vi "game.vi"() -> ()   [LabVIEW 2016]
panel:
  in  "ModeIsSetting":bool=TRUE
  in  "Tab Control":enum32{"Game", "Settings", "How to Play"}(tab)
  out "Target LED Ready":bool
  out "Current Player":string
  out "?":bool[](array[boolean])
  out "?":bool[](array[boolean])
  out "Players":string[](array[string])
  out "Scores":i32[](array[numeric])
  out "Current Player":i32
  out "Current LED":i32
  out "LED Ready":bool
  out "Target LED":i32
  out "player ready":bool=TRUE
  in  "stop":bool
  in  "RESET":bool
  out "Score":string
  in  "current duration":u32
  in  "Start The Game":bool
  in  "Game Mode":enum16{"Easy", "Hard", "Very Hard"}(ring)
  in  "LED count":i32=10
  in  "starting LED\nduration":u32=100
  in  "Player count":i32=2
  in  "Player prefix":string="Player"
  in  "duration decrease":u32=20
  in  "min duration":u32=60
  in  "Target Led duration":i32=1000
  out "Blank LEDs":bool[](array[boolean])
  # "L  E  D     G  A  M  E  !"
  # "Game Settings"
  # "H o w    t o    P l a y    ?"
  # "1 - Set the parameters in the settings tab as you wish\n\n2 - By clicking on the stop button you can stop the circle LED in the red state. The rectangle red LED shows on which led you should click on the stop button.\n\n3 - The more closer you stop the red circle LED to red rectangle LED, the more points you achieve to gain.\n\n4 - Be carefull, as the game moves on, the the LEDs will start to turn on and off more quickly according to the settings you choose.\n\n5 - Modes\nEasy: The target LED does not move.\nHard: The target LED also moves with the duration you set in the settings tab.\nVery Hard: The target LED moves randomly, being talented is not enough you should also be lucky ! \n\n\n                                                           Have Fun !"
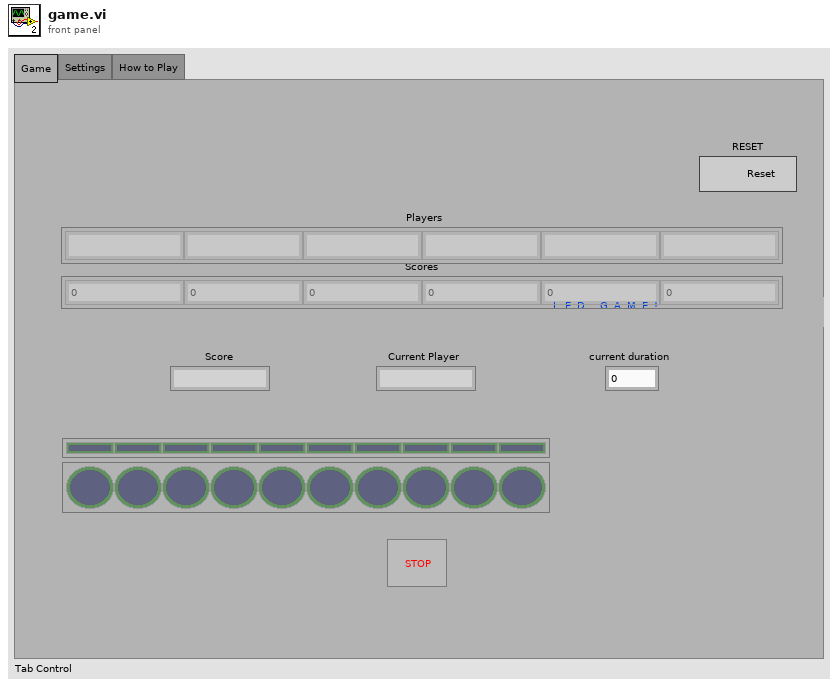
[diagram p1: front panel]
types:
  T1 = enum8{"Enabled", "Disabled", "Disabled and Grayed Out"}
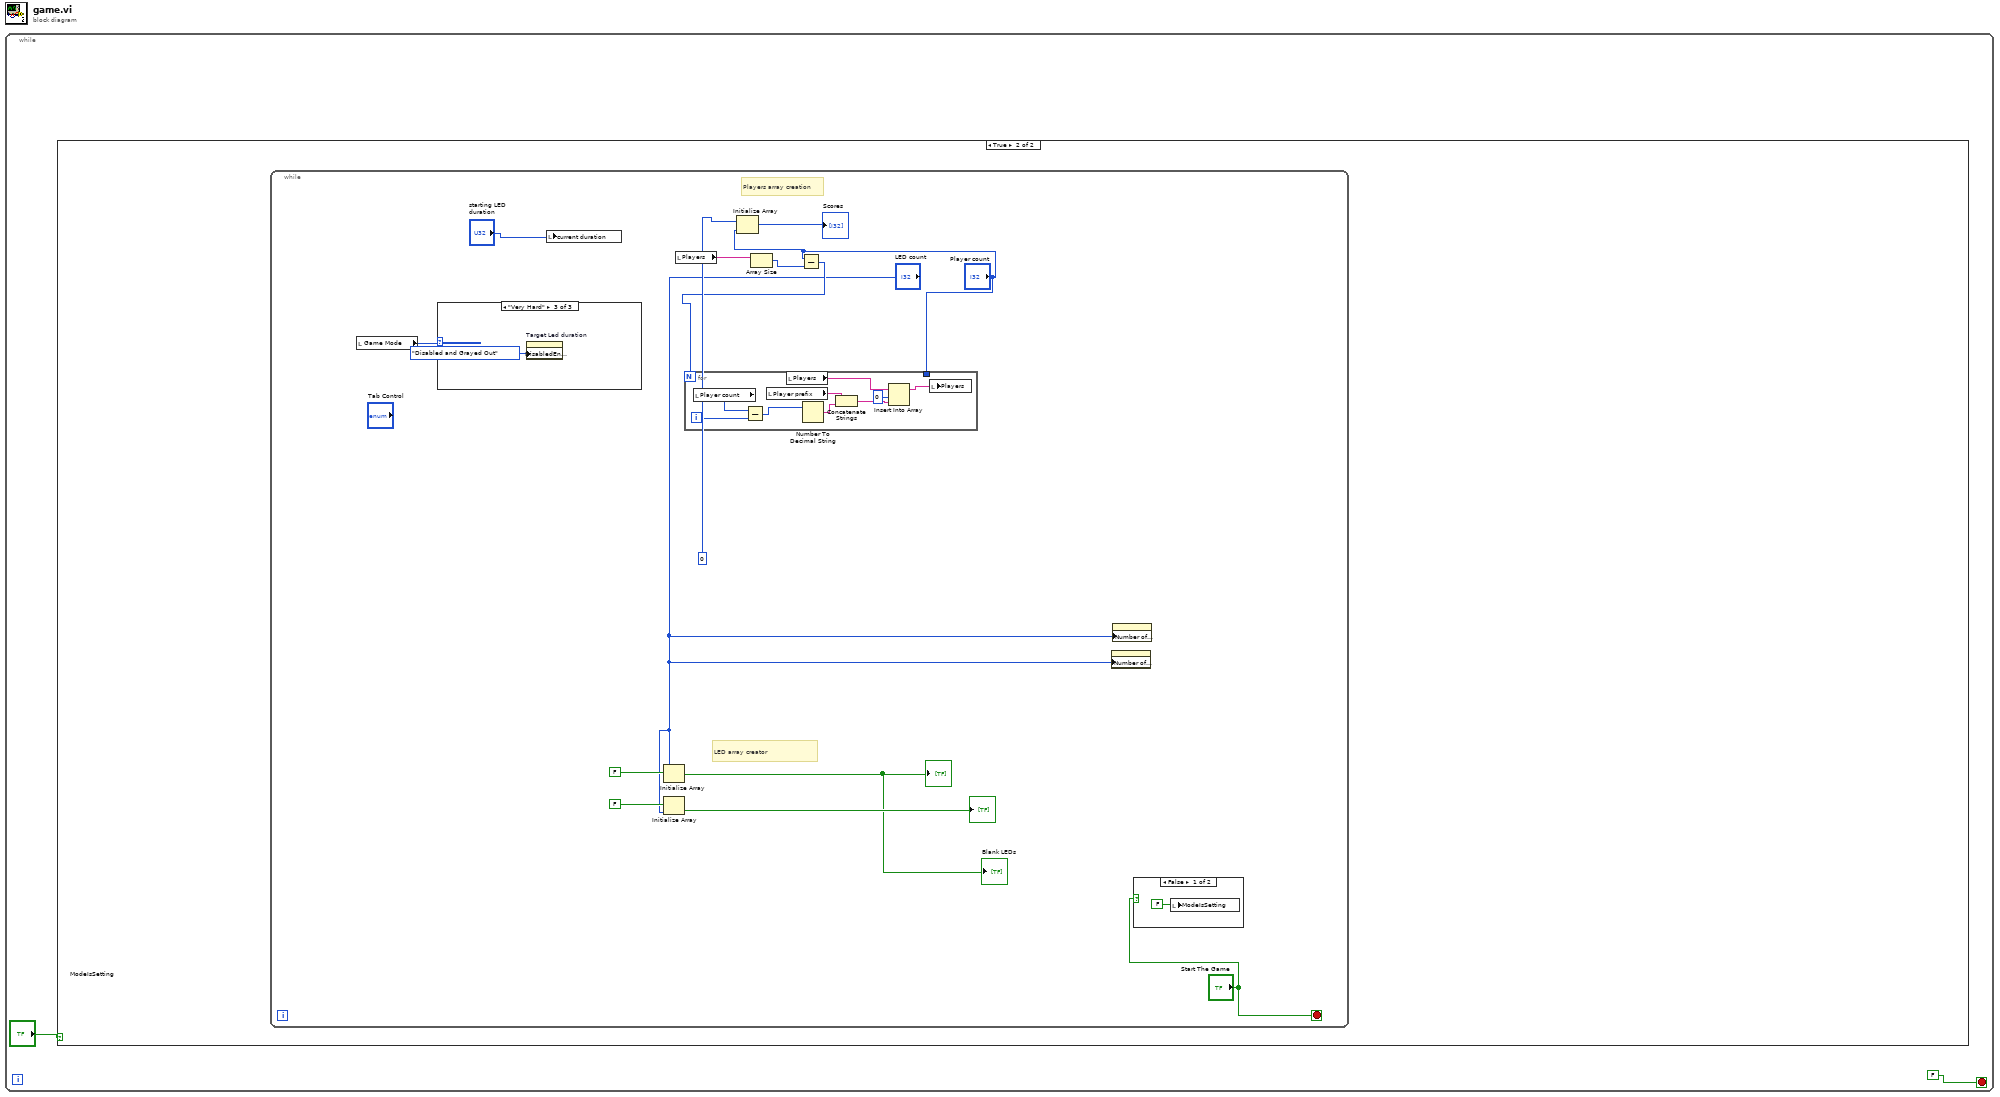
[diagram p0: block diagram]
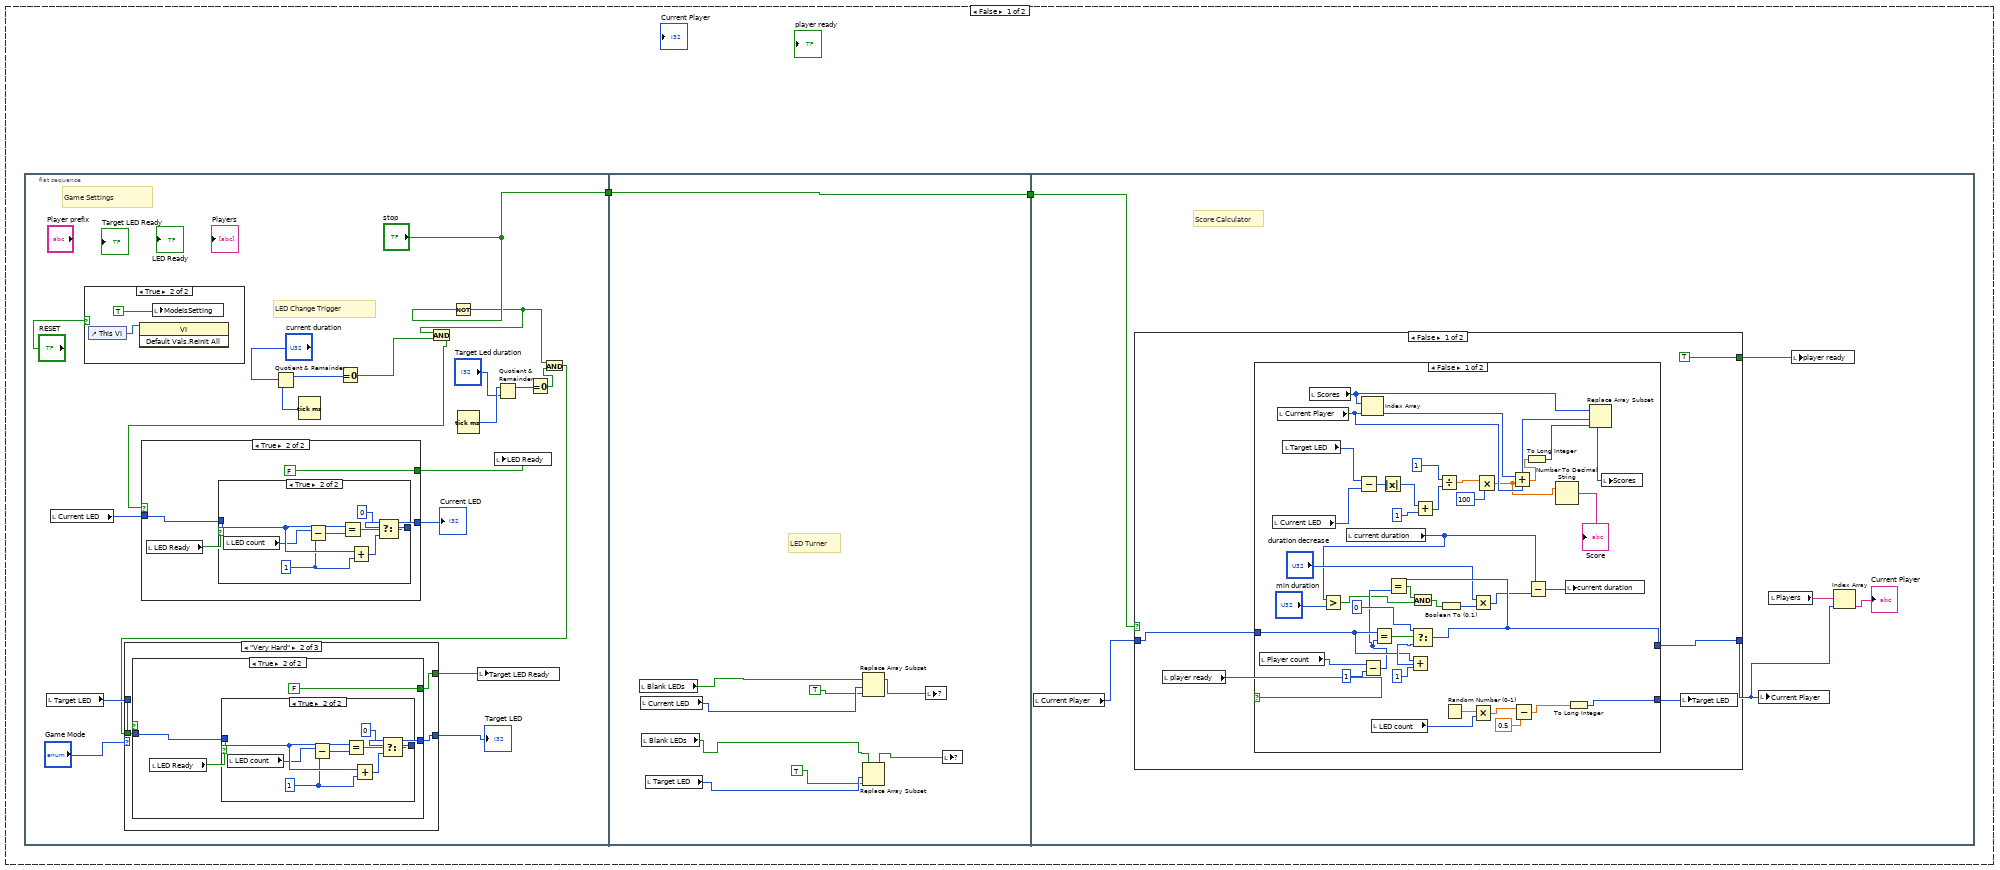
[diagram p2: hidden frame]
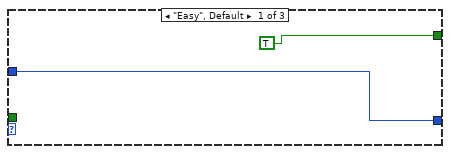
[diagram p3: hidden frame]
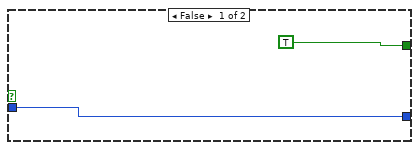
[diagram p4: hidden frame]
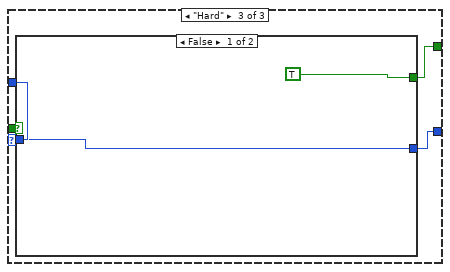
[diagram p6: hidden frame]
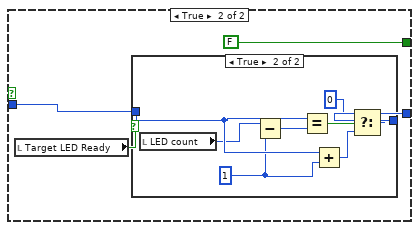
[diagram p7: hidden frame]
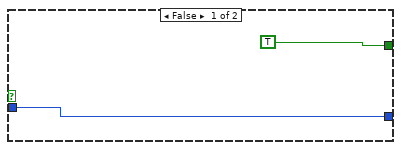
[diagram p10: hidden frame]
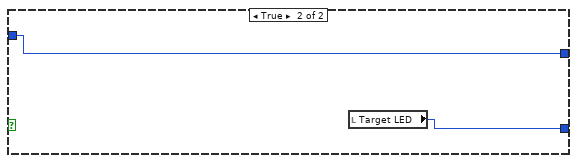
[diagram p12: hidden frame]
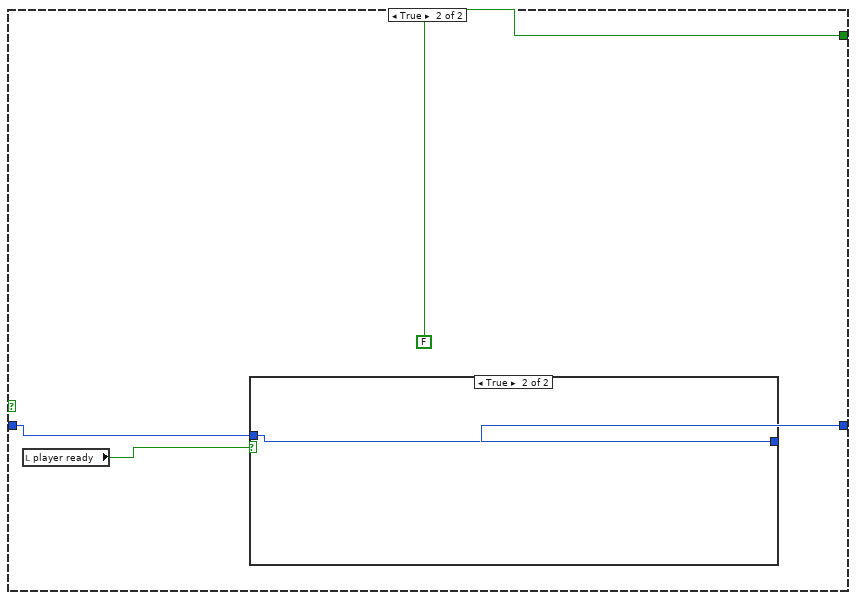
[diagram p13: hidden frame]
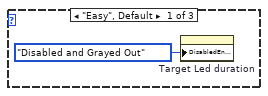
[diagram p16: hidden frame]
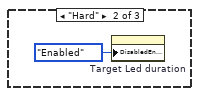
[diagram p17: hidden frame]
diagram:
  n1 = while {
    stop <- FALSE stop-if-true
    n2 = case shown="True" "ModeIsSetting" {
      frame False {
        n3 = flat-sequence {
          tunnel: ["stop"] -> w4
          tunnel: w4 -> [w84]
          tunnel: [w84] -> w3
          tunnel: w3 -> [w94]
          frame #0 {
            # "LED Change Trigger"
            # "Game Settings"
            n4 = local read "Target LED"() -> (w13:i32)
            n5 = local read "Current LED"() -> (w22:i32)
            n6 = case shown="True" "RESET" {
              frame False {
              }
              frame True {
                n7 = control-ref of="This VI"() -> (w66:refnum<vi>)
                n8 = invoke class="VI" method="Default Vals.Reinit All"(reference=w66) -> ()  [unwired: 2 in, 3 out]
                n9 = local write "ModeIsSetting"(TRUE) -> ()
              }
            }
            n10 = Tick Count (ms)() -> (millisecond timer value=w24:u32)
            n11 = Quotient & Remainder(x=w24, y="current duration") -> (x-y*floor(x/y)=w23:u32)  [unwired: 1 out]
            n12 = Equal To 0?(x=w23) -> (x = 0?=w19:bool)
            n13 = Not(x="stop") -> (.not. x?=w7:bool)
            n14 = And(x=w7, y=w19) -> (x .and. y?=w12:bool)
            n15 = case shown="True" w12 {
              tunnel: w22 -> [w68 w72]
              tunnel: [w68 w71] -> w21
              tunnel: [TRUE FALSE] -> w20
              frame False {
              }
              frame True {
                n16 = local read "LED Ready"() -> (w69:bool)
                n17 = case shown="True" w69 {
                  tunnel: w72 -> [w73 w81]
                  tunnel: [w73 w80] -> w71
                  frame False {
                  }
                  frame True {
                    w74 = 1
                    n18 = local read "LED count"() -> (w75:i32)
                    n19 = Subtract(x=w75, y=w74) -> (x-y=w76:i32)
                    n20 = Equal?(x=w81, y=w76) -> (x = y?=w79:bool)
                    n21 = Add(x=w81, y=w74) -> (x+y=w77:i32)
                    n22 = Select(t=0, s=w79, f=w77) -> (s? t:f=w80:i32)
                  }
                }
              }
            }
            "Current LED" <- w21
            n23 = Tick Count (ms)() -> (millisecond timer value=w11:u32)
            n24 = local write "LED Ready"(w20) -> ()
            n25 = Quotient & Remainder(x=w11, y="Target Led duration") -> (x-y*floor(x/y)=w9:u32)  [unwired: 1 out]
            n26 = Equal To 0?(x=w9) -> (x = 0?=w8:bool)
            n27 = And(x=w7, y=w8) -> (x .and. y?=w6:bool)
            n28 = case shown="\"Very Hard\"" "Game Mode" {
              tunnel: [w26 w29 w48] -> w14
              tunnel: w13 -> [w26 w27 w49]
              tunnel: w6 -> [_ w28 w47]
              tunnel: [TRUE w30 w46] -> w5
              frame "Easy", Default {
              }
              frame "Very Hard" {
                n29 = case shown="True" w28 {
                  tunnel: w27 -> [w32 w36]
                  tunnel: [w32 w35] -> w29
                  tunnel: [TRUE FALSE] -> w30
                  frame False {
                  }
                  frame True {
                    n30 = local read "LED Ready"() -> (w33:bool)
                    n31 = case shown="True" w33 {
                      tunnel: w36 -> [w37 w45]
                      tunnel: [w37 w44] -> w35
                      frame False {
                      }
                      frame True {
                        w38 = 1
                        n32 = local read "LED count"() -> (w39:i32)
                        n33 = Subtract(x=w39, y=w38) -> (x-y=w40:i32)
                        n34 = Equal?(x=w45, y=w40) -> (x = y?=w43:bool)
                        n35 = Add(x=w45, y=w38) -> (x+y=w41:i32)
                        n36 = Select(t=0, s=w43, f=w41) -> (s? t:f=w44:i32)
                      }
                    }
                  }
                }
              }
              frame "Hard" {
                n37 = case shown="False" w47 {
                  tunnel: w49 -> [w51 w55]
                  tunnel: [w51 w54] -> w48
                  tunnel: [TRUE FALSE] -> w46
                  frame False {
                  }
                  frame True {
                    n38 = local read "Target LED Ready"() -> (w52:bool)
                    n39 = case shown="True" w52 {
                      tunnel: w55 -> [w56 w64]
                      tunnel: [w56 w63] -> w54
                      frame False {
                      }
                      frame True {
                        w57 = 1
                        n40 = local read "LED count"() -> (w58:i32)
                        n41 = Subtract(x=w58, y=w57) -> (x-y=w59:i32)
                        n42 = Equal?(x=w64, y=w59) -> (x = y?=w62:bool)
                        n43 = Add(x=w64, y=w57) -> (x+y=w60:i32)
                        n44 = Select(t=0, s=w62, f=w60) -> (s? t:f=w63:i32)
                      }
                    }
                  }
                }
              }
            }
            "Target LED" <- w14
            n45 = local write "Target LED Ready"(w5) -> ()
          }
          frame #1 {
            # "LED Turner"
            n46 = local read "Blank LEDs"() -> (w85:bool[])
            n47 = local read "Current LED"() -> (w86:i32)
            n48 = local read "Blank LEDs"() -> (w90:bool[])
            n49 = local read "Target LED"() -> (w88:i32)
            n50 = Replace Array Subset(array=w85, new element=TRUE, index=w86) -> (w87:bool[])
            n51 = Replace Array Subset(array=w90, new element=TRUE, index=w88) -> (w89:bool[])
            n52 = local write item#?(w87) -> ()
            n53 = local write item#11(w89) -> ()
          }
          frame #2 {
            # "Score Calculator"
            n54 = local read "Current Player"() -> (w96:i32)
            n55 = case shown="False" w94 {
              tunnel: [TRUE FALSE] -> w95
              tunnel: [w99 w147] -> w92
              tunnel: w96 -> [w98 w145]
              frame False {
                n56 = local read "player ready"() -> (w100:bool)
                n57 = case shown="False" w100 {
                  tunnel: [w114 w144] -> w99
                  tunnel: w98 -> [w133 w144]
                  tunnel: [w132 w143] -> w97
                  frame False {
                    n58 = local read "Player count"() -> (w115:i32)
                    n59 = local read "Current LED"() -> (w130:i32)
                    n60 = local read "Current Player"() -> (w123:i32)
                    n61 = local read "Target LED"() -> (w131:i32)
                    n62 = local read "Scores"() -> (w124:i32[])
                    n63 = local read "current duration"() -> (w108:u32)
                    n64 = Greater?(x=w108, y="min duration") -> (0:w102:bool)
                    n65 = Subtract(x=w131, y=w130) -> (x-y=w129:i32)
                    n66 = Index Array(array=w124, index=w123) -> (element=w125:i32)
                    n67 = Subtract(x=w115, y=1) -> (x-y=w109:i32)
                    n68 = local read "LED count"() -> (w140:i32)
                    n69 = Equal?(x=w133, y=w109) -> (x = y?=w104:bool)
                    n70 = Absolute Value(x=w129) -> (abs(x)=w120:i32)
                    n71 = Add(x=w133, y=1) -> (x+y=w137:i32)
                    n72 = Select(t=0, s=w104, f=w137) -> (s? t:f=w114:i32)
                    n73 = Equal?(x=w114, y=w109) -> (x = y?=w105:bool)
                    n74 = And(x=w105, y=w102) -> (x .and. y?=w106:bool)
                    n75 = Add(x=w120, y=1) -> (x+y=w118:i32)
                    n76 = Divide(x=1, y=w118) -> (x/y=w127:dbl)
                    n77 = Boolean To (0,1)(Boolean=w106) -> (0, 1=w113:i16)
                    n78 = Random Number (0-1)() -> (number: 0 to 1=w141:dbl)
                    n79 = Multiply(x="duration decrease", y=w113) -> (x*y=w111:u32)
                    n80 = Multiply(x=w141, y=w140) -> (x*y=w139:dbl)
                    n81 = Multiply(x=w127, y=100) -> (x*y=w103:dbl)
                    n82 = Add(x=w125, y=w103) -> (x+y=w122:dbl)
                    n83 = Subtract(x=w139, y=0.5) -> (x-y=w142:dbl)
                    n84 = To Long Integer(number=w122) -> (32bit integer=w117:i32)
                    n85 = Subtract(x=w108, y=w111) -> (x-y=w110:u32)
                    n86 = Number To Decimal String(number=w103) -> (decimal integer string=→"Score":string)  [unwired: 1 in]
                    n87 = local write "current duration"(w110) -> ()
                    n88 = To Long Integer(number=w142) -> (32bit integer=w132:i32)
                    n89 = Replace Array Subset(array=w124, new element=w117, index=w123) -> (w121:i32[])
                    n90 = local write "Scores"(w121) -> ()
                  }
                  frame True {
                    n91 = local read "Target LED"() -> (w143:i32)
                  }
                }
                n92 = local write "Target LED"(w97) -> ()
              }
              frame True {
                n93 = local read "player ready"() -> (w146:bool)
                n94 = case shown="True" w146 {
                  tunnel: [w149 w150] -> w147
                  tunnel: w145 -> [w149 w150]
                  frame False {
                  }
                  frame True {
                  }
                }
              }
            }
            n95 = local write "Current Player"(w92) -> ()
            n96 = local read "Players"() -> (w93:string[])
            n97 = local write "player ready"(w95) -> ()
            n98 = Index Array(array=w93, index=w92) -> (element=→"Current Player":string)
          }
        }
      }
      frame True {
        n99 = while {
          stop <- "Start The Game" stop-if-true
          # "Players array creation"
          # "LED array creator"
          n100 = local read "Game Mode"() -> (w152:enum16{"Easy", "Hard", "Very Hard"})
          n101 = case shown="\"Very Hard\"" w152 {
            frame "Easy", Default {
              n102 = property on="Target Led duration" class="DigNum (strict)"("DisabledEnum"=T1."Disabled and Grayed Out" ("Disabled")) -> ()  [unwired: 2 in, 2 out]
            }
            frame "Hard" {
              n103 = property on="Target Led duration" class="DigNum (strict)"("DisabledEnum"=T1."Enabled" ("Disabled")) -> ()  [unwired: 2 in, 2 out]
            }
            frame "Very Hard" {
              n104 = property on="Target Led duration" class="DigNum (strict)"("DisabledEnum"=T1."Disabled and Grayed Out" ("Disabled")) -> ()  [unwired: 2 in, 2 out]
            }
          }
          n105 = local write "current duration"("starting LED\nduration") -> ()
          n106 = Initialize Array(FALSE ("Boolean"), "LED count") -> (→"?" →"Blank LEDs":bool[])
          n107 = Initialize Array(FALSE ("Boolean"), "LED count") -> (→"?":bool[])
          n108 = local read "Players"() -> (w157:string[])
          n109 = Initialize Array(0, "Player count") -> (→"Scores":i32[])
          n110 = Array Size(array=w157) -> (size(s)=w158:i32)
          n111 = Subtract(x="Player count", y=w158) -> (x-y=w159:i32)
          n112 = for {
            N: w159 -> [_]
            tunnel: "Player count" -> [_]
            i -> [w169]
            n113 = local read "Player count"() -> (w170:i32)
            n114 = Subtract(x=w170, y=w169) -> (x-y=w171:i32)
            n115 = local read "Player prefix"() -> (w177:string)
            n116 = local read "Players"() -> (w175:string[])
            n117 = Number To Decimal String(number=w171) -> (decimal integer string=w173:string)  [unwired: 1 in]
            n118 = Concatenate Strings(w177, w173) -> (w176:string)
            n119 = Insert Into Array(array=w175, index=0, new element=w176) -> (w172:string[])
            n120 = local write "Players"(w172) -> ()
          }
          n121 = property class="Arr (strict)"("Number of Columns"="LED count") -> ()  [unwired: 2 in, 2 out]
          n122 = property class="Arr (strict)"("Number of Columns"="LED count") -> ()  [unwired: 2 in, 2 out]
          n123 = case shown="False" "Start The Game" {
            frame False {
              n124 = local write "ModeIsSetting"(FALSE) -> ()
            }
            frame True {
            }
          }
        }
      }
    }
  }
